vi "Initialization VI.vi"(8 "error in (no error)":errorcluster, 10 "Custom XML":string, 11 "Device Item Ref in":T1 format="%.0x") -> (0 "error out":errorcluster, 3 "Device Item Ref out":T1 format="%.0x")   [LabVIEW 2015, in "Development Tools Examples System Explorer.lvlib"]
uses:
  Development Tools Examples System Explorer.lvlib
  <vilib>/NI Veristand/Custom Device API/Custom Device Item Ref.ctl
  <vilib>/Utility/config.llb/Read Key (Boolean).vi
  Shared/Constants.vi
  <vilib>/NI Veristand/Custom Device API/Custom Device API.lvlib
  <vilib>/Utility/config.llb/NI_LVConfig.lvlib
  Shared/Development Tools Examples Shared.lvlib
panel:
  out "Errors":string="6b16e173-82d5-42e9-a892-d10f89a4f636"
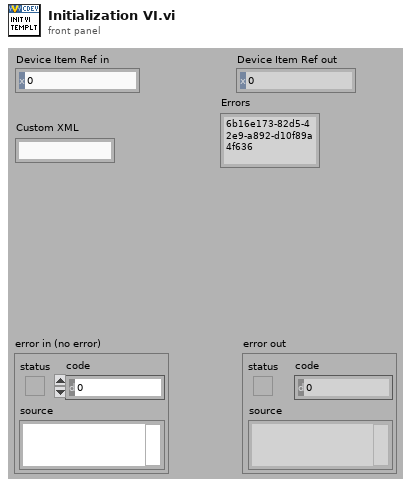
[diagram p1: front panel]
types:
  T1 = typedef "Custom Device API.lvlib/Custom Device Item Ref.ctl" = u64
  T2 = typedef "NI_LVConfig.lvlib/Config Data RefNum.ctl" = refnum<k1>
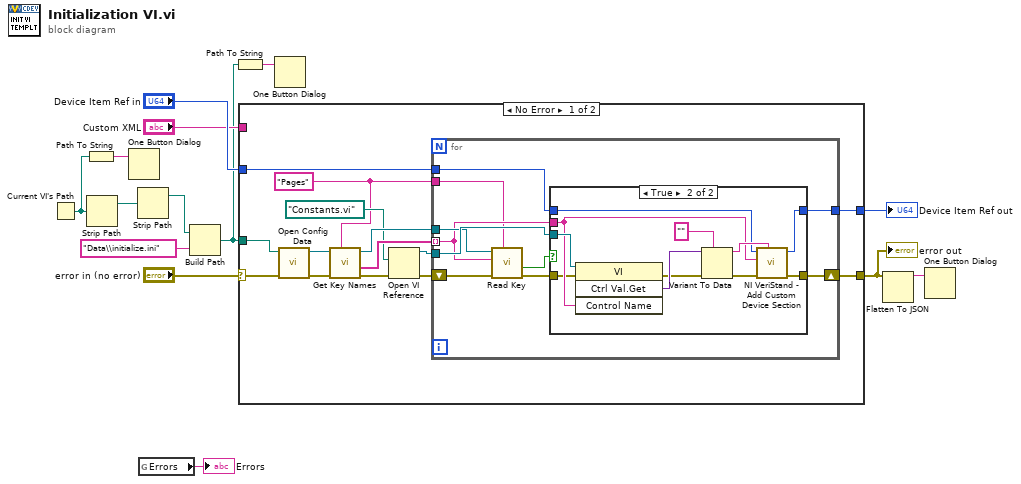
[diagram p0: block diagram]
diagram:
  n1 = Current VI's Path() -> (path=w7:path)
  n2 = Path To String(path=w7) -> (string=w8:string)
  n3 = Strip Path(path=w7) -> (stripped path=w6:path)  [unwired: 1 out]
  n4 = One Button Dialog(message=w8) -> ()  [unwired: 1 in, 1 out]
  n5 = Strip Path(path=w6) -> (stripped path=w5:path)  [unwired: 1 out]
  n6 = global read "Constants.vi" "Errors"() -> (→"Errors":string)
  n7 = Build Path(base path=w5, name or relative path="Data\\initialize.ini") -> (appended path=w2:path)
  n8 = Path To String(path=w2) -> (string=w3:string)
  n9 = case shown="No Error" "error in (no error)" {
    selector: "error in (no error)" -> [w22 w53]
    tunnel: [w18 w53] -> w10
    tunnel: [w23 w52] -> w13
    tunnel: "Device Item Ref in" -> [w24 w52]
    tunnel: "Custom XML" -> [_ _]
    tunnel: w2 -> [w15 _]
    frame No Error {
      w16 = "Pages" ("section")
      n10 = call <vilib>:"Open Config Data.vi"("error in (no error)"=w22, "configuration file path"=w15) -> ("error out"=w21:errorcluster, "refnum"=w28:T2)  [unwired: 7 in, 1 out]
      n11 = call <vilib>:"Get Key Names.vi"("section"=w16, "error in (no error)"=w21, "refnum"=w28) -> ("error out"=w20:errorcluster, "key names"=w27:string[], "refnum out"=w25:T2)  [unwired: 5 in, 1 out]
      n12 = Open VI Reference(vi path=path "Constants.vi", error in (no error)=w20) -> (vi reference=w26:refnum<vi>, error out=w19:errorcluster)  [unwired: 4 in]
      n13 = for {
        tunnel: w27 -> [w36] mode=indexing
        tunnel: w26 -> [w38]
        tunnel: w25 -> [w37]
        tunnel: w24 -> [w34]
        tunnel: [w33] -> w23
        tunnel: w16 -> [w29]
        shift-right: [w30] -> w18
        shift-left: w19 -> [w32]
        n14 = call-poly <vilib>:"Read Key.vi"("section"=w29, "error in (no error)"=w32, "key"=w36, "refnum"=w37) -> ("error out"=w31:errorcluster, "value"=w35:bool)  [unwired: 4 in, 2 out]
        n15 = case shown="True" w35 {
          tunnel: w38 -> [_ w49]
          tunnel: w36 -> [_ w47]
          tunnel: w34 -> [w40 w46]
          tunnel: [w40 w45] -> w33
          tunnel: w31 -> [w39 w44]
          tunnel: [w39 w41] -> w30
          frame False {
          }
          frame True {
            n16 = invoke class="VI" method="Ctrl Val.Get"(reference=w49, error in=w44, "Control Name"=w47) -> (error out=w43:errorcluster, "Get Control Value Variant"=w51:variant)  [unwired: 1 in, 2 out]
            n17 = Variant To Data(error in=w43, type="", Variant=w51) -> (data=w48:string, error out=w42:errorcluster)
            n18 = call <vilib>:"NI VeriStand - Add Custom Device Section.vi"("GUID (Default Section)"=w48, "error in (no error)"=w42, "Section Name"=w47, "Parent Ref in"=w46) -> ("error out"=w41:errorcluster, "Parent Ref out"=w45:T1)  [unwired: 4 in, 2 out]
          }
        }
      }
    }
    frame Error {
    }
  }
  "error out" <- w10
  "Device Item Ref out" <- w13
  n19 = One Button Dialog(message=w3) -> ()  [unwired: 1 in, 1 out]
  n20 = Flatten To JSON(anything=w10) -> (JSON string=w9:string)  [unwired: 2 in, 1 out]
  n21 = One Button Dialog(message=w9) -> ()  [unwired: 1 in, 1 out]
